vi "Initialize.vi"(11 "error in (no error)":errorcluster) -> (4 "GEA2 Reference Out":refnum<k24>, 8 "Pass/Fail?":bool, 10 "Report Text":string, 15 "error out":errorcluster)   [LabVIEW 2016]
uses:
  C:/Automation/DLLs/PC Dot Net/GeaCommunication.dll
  Automation/DLLs/PC Dot Net/GeaCommunication.dll
  Q:/Common/LabVIEW GEA2 Toolkit/LabVIEW_GEA2_Toolkit.lvlibp/type defs/Source_Destination.ctl
  Q:/Common/LabVIEW GEA2 Toolkit/LabVIEW_GEA2_Toolkit.lvlibp
  Q:/Automation/Product Specific/Clothes Care/TL27/Projects/TL27.lvlib
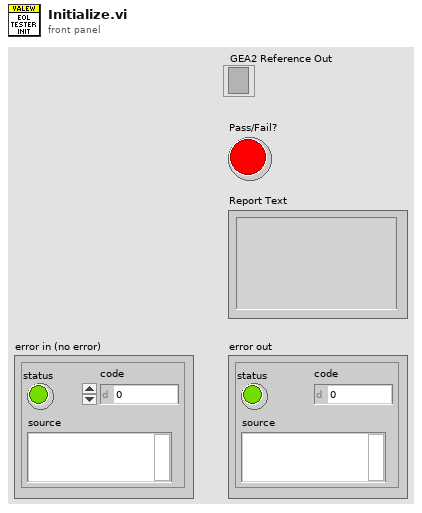
[diagram p1: front panel]
types:
  T1 = typedef "LabVIEW_GEA2_Toolkit.lvlibp/Source_Destination.ctl" = cluster{"Source":u8, "Destination":u8}
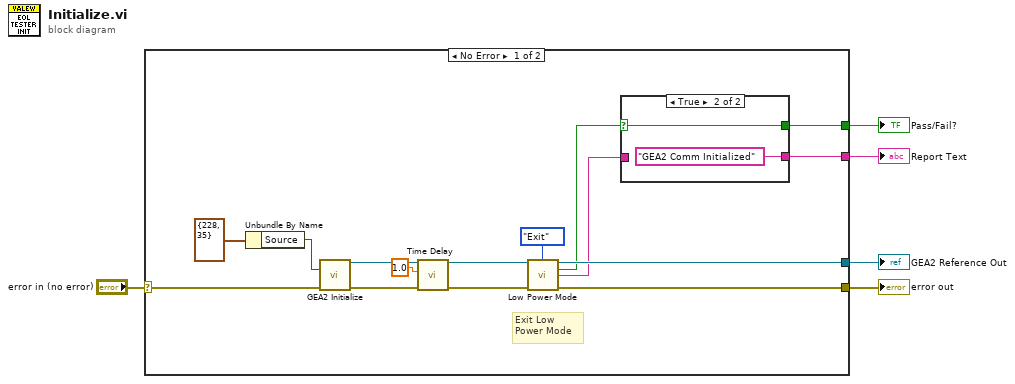
[diagram p0: block diagram]
diagram:
  n1 = case shown="No Error" "error in (no error)" {
    selector: "error in (no error)" -> [w6 w24]
    tunnel: [w15 w24] -> w5
    tunnel: [w14 _] -> w4
    tunnel: [w11 _] -> w3
    tunnel: [w10 _] -> w2
    frame No Error {
      # "Exit Low\nPower Mode"
      n2 = Unbundle By Name(T1 {"Source"=228, "Destination"=35} ("GEA Inputs")) -> ("Source"=w18:u8)
      n3 = call "GEA2 Initialize.vi"("Source Address"=w18, "error in"=w6) -> ("GEA2 Reference Out"=w17:refnum<k24>, "error out"=w16:errorcluster)  [unwired: 11 in, 1 out]
      n4 = call "Time Delay"("error in (no error)"=w16, "Delay Time (s)"=1.0) -> ("error out"=w8:errorcluster)  [unwired: 9 in]
      n5 = call "Low Power Mode.vi"("GEA2 Reference In"=w17, "Action"=enum16{"Enter", "Exit"}."Exit", "Error In"=w8) -> ("GEA2 Reference Out"=w14:refnum<k24>, "Pass/Fail?"=w12:bool, "Report Text"=w9:string, "Error Out"=w15:errorcluster)  [unwired: 9 in]
      n6 = case shown="True" w12 {
        selector: w12 -> [w20 w23]
        tunnel: [w20 w23] -> w11
        tunnel: [w21 "GEA2 Comm Initialized"] -> w10
        tunnel: w9 -> [w21 _]
        frame False {
        }
        frame True {
        }
      }
    }
    frame Error {
    }
  }
  "error out" <- w5
  "GEA2 Reference Out" <- w4
  "Pass/Fail?" <- w3
  "Report Text" <- w2
